vi "Extract Varient.vi"(7 "Copy":bool caption="Copy data instead of extracting", 8 "error in (no error)":errorcluster, 11 "Message":refnum<class "VarMessage.lvclass">) -> (0 "error out":errorcluster, 1 "Varient":variant, 2 "Label":string, 3 "Message (data extracted)":refnum<class "VarMessage.lvclass">)   [LabVIEW 2011, in "Messenging.lvlib" / "VarMessage.lvclass"]
uses:
  VarMessage.lvclass
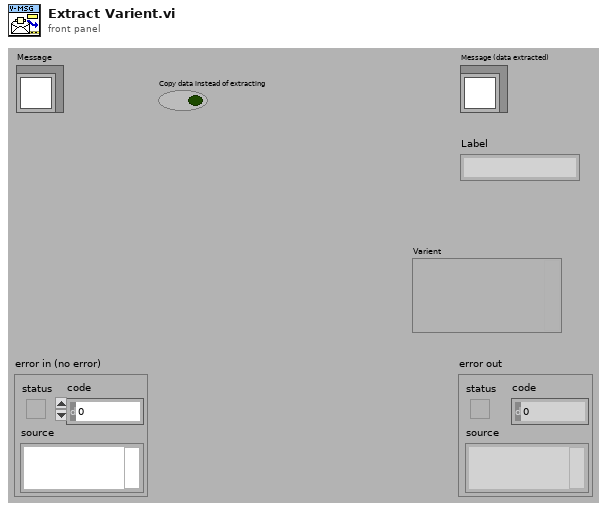
[diagram p1: front panel]
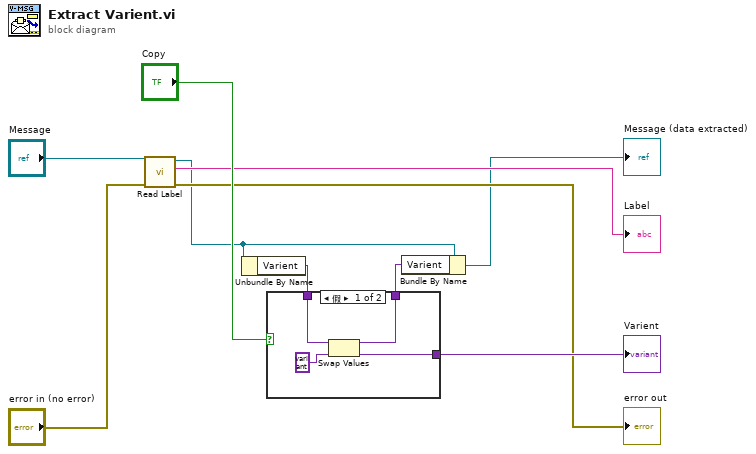
[diagram p0: block diagram]
diagram:
  n1 = call-dynamic "Read Label.vi"("error in (no error)"="error in (no error)", "Message"="Message") -> ("error out"=→"error out":errorcluster, "Label"=→"Label":string, "Message"=w2:refnum<class "VarMessage.lvclass">)  [unwired: 7 out]
  n2 = Unbundle By Name(w2) -> ("Varient"=w6:variant)
  n3 = case shown="假" "Copy" {
    tunnel: w6 -> [w14 w15]
    tunnel: [w13 w15] -> w5
    tunnel: [w12 w15] -> w10
    frame False {
      n4 = Swap Values(12:w14, 14:variant ("Varient")) -> (1:w13:variant, 3:w12:variant)  [unwired: 1 out]
    }
    frame True {
    }
  }
  "Varient" <- w10
  n5 = Bundle By Name(cluster=w2, "Varient"=w5) -> (→"Message (data extracted)":refnum<class "VarMessage.lvclass">)
